vi "util.log.compress.vi"(11 "Log Cluster in":T3 {"clk" format="%#.3f"}) -> (2 "Proc Name":string, 3 "Compact Report":T1 {"clk" format="%#.1f"})   [LabVIEW 2024]
uses:
  controls/typeEngineLogCluster.ctl
  controls/type.StepFunction.ctl
  controls/UiCompactReport.ctl
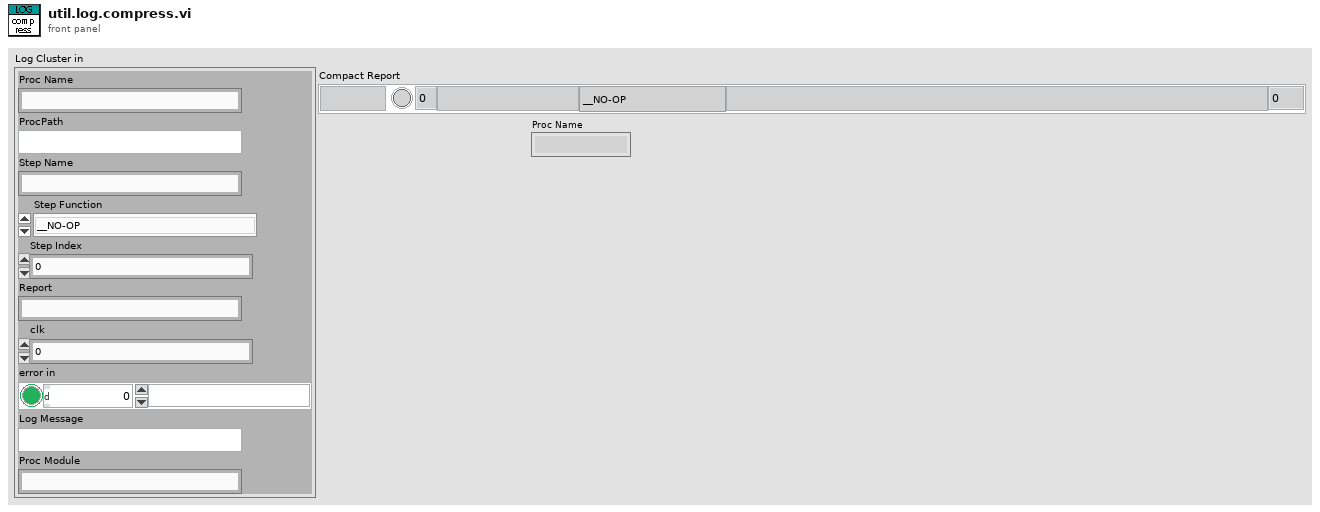
[diagram p1: front panel]
types:
  T1 = typedef "UiCompactReport.ctl" = cluster{"ErrorFlag":bool, "idx":i32, "Step Name":string, "Step Function":T2, "Report":string, "clk":dbl, "Proc":string}
  T2 = typedef "type.StepFunction.ctl" = enum16{"__NO-OP", "_DELAY_LOAD", "_DELAY_COMPARE", "_JUMP", "_COMPLETE", "_COMPARE", "_LOG_MESSAGE", "_LOG_LAST_REPORT", "_SCHEDULE", "_SCHED_DAILY", "CLK_COMPARE", "PROC_START", "PROC_STOP", "PROC_LOAD", "PROC_COMPLETION_CHECK", "PROC_COMPLETION_LOAD", "_IO_READ", "_IO_READ_MANY", "_IO_WRITE", "_IO_WRITE_BY_REG", "_IO_GET_OUTPUT", "_OCS_CHECK", "_OCS_RECORD", "_GET_RH", "_GET_ACC_UV", "_GET_WD", "_GET_WS", "_REC_DELETE", "_REC_MOVE", "_REC_COPY", "_IRR_CHECK", "UNIT_CHECK", "UNIT_SAMPLE", "UNIT_DOSE"}
  T3 = typedef "typeEngineLogCluster.ctl" = cluster{"Proc Name":string, "ProcPath":string, "Step Name":string, "Step Function":T2, "Step Index":i32, "Report":string, "clk":dbl, "error in":errorcluster, "Log Message":string, "Proc Module":string}
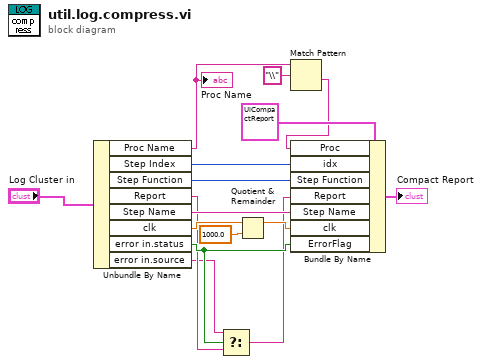
[diagram p0: block diagram]
diagram:
  n1 = Unbundle By Name("Log Cluster in") -> ("Proc Name"=w1:string, "Step Index"=w12:i32, "Step Function"=w11:T2, "Report"=w6:string, "Step Name"=w13:string, "clk"=w10:dbl, "error in.status"=w7:bool, "error in.source"=w4:string)
  "Proc Name" <- w1
  n2 = Select(t=w4, s=w7, f=w6) -> (s? t:f=w5:string)
  n3 = Quotient & Remainder(x=w10, y=1000.0) -> (x-y*floor(x/y)=w8:dbl)  [unwired: 1 out]
  n4 = Match Pattern(string=w1, regular expression="\\") -> (after substring=w2:string)  [unwired: 1 in, 3 out]
  n5 = Bundle By Name(cluster=T1 {"ErrorFlag"=FALSE, "idx"=0, "Step Name"="", "Step Function"=enum."__NO-OP", "Report"="", "clk"=0.0, "Proc"=""} ("compact report 2"), "Proc"=w2, "idx"=w12, "Step Function"=w11, "Report"=w5, "Step Name"=w13, "clk"=w8, "ErrorFlag"=w7) -> (→"Compact Report":T1)
